vi "Day 6.vi"() -> ()   [LabVIEW 2019]
panel:
  out "Largest Finite Area":i16
  out "Filtered Closest Point Indices":i32[][](array[numeric])
  out "Closest Point Indices":i32[][](array[numeric])
  out "Distances":i32[][][](array[numeric])
  out "Min Values":i32[](array[numeric])
  out "Max Values":i32[](array[numeric])
  out "Coordinates":i32[][](array[numeric])
  in  "Error In":errorcluster
  in  "Use Example Input":bool
  in  "Example Input":string="1, 1\n1, 6\n8, 3\n3, 4\n5, 5\n8, 9\n"
  in  "Relative Path to Input File":string="Day 6\\Day 6 Raw Input.txt"
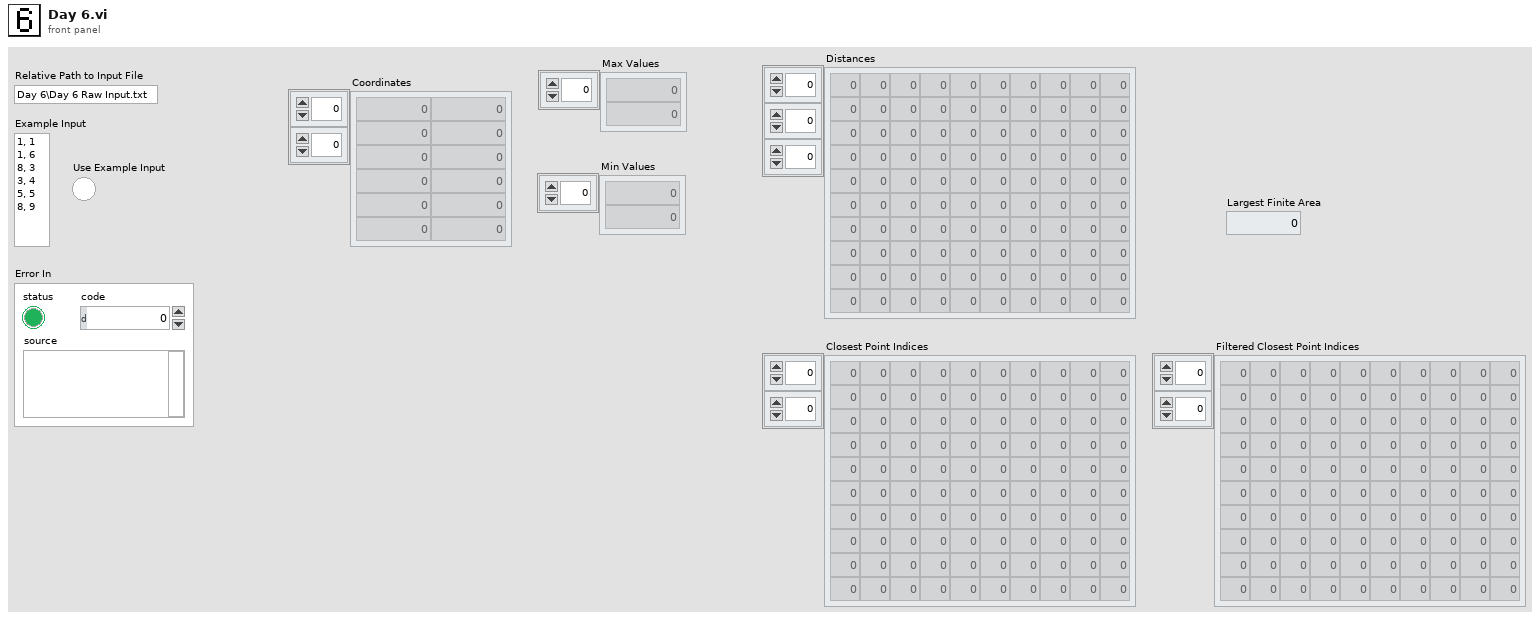
[diagram p1: front panel]
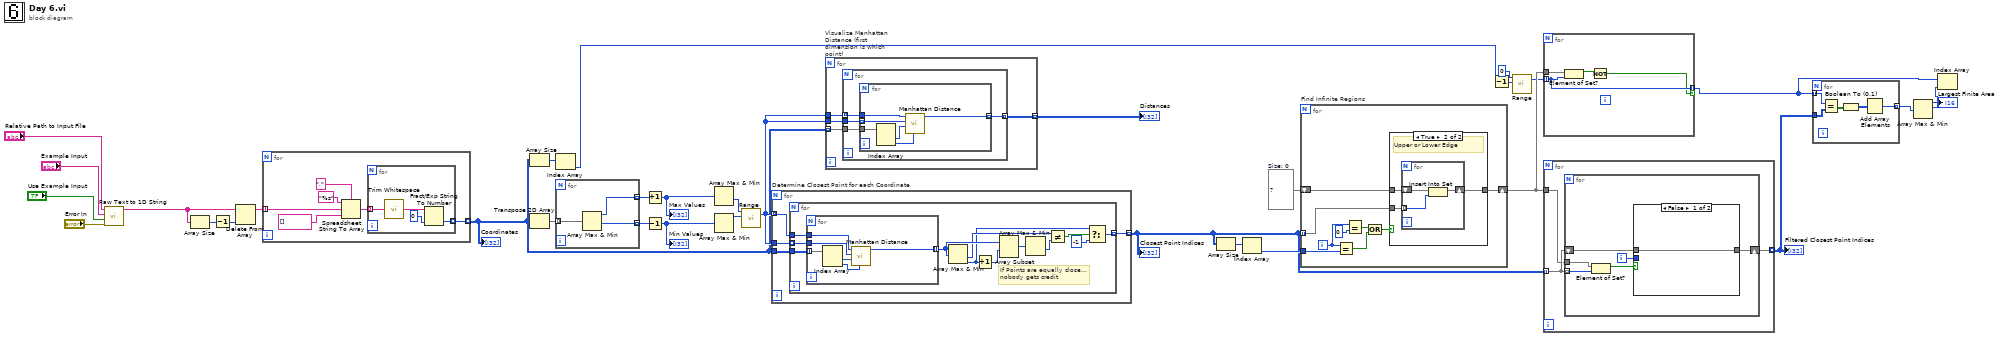
[diagram p0: block diagram]
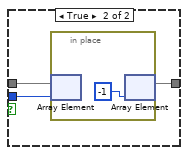
[diagram p2: hidden frame]
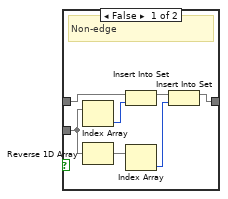
[diagram p3: hidden frame]
diagram:
  w14 = set{i32} {}  # Size: 0
  n1 = call "Raw Text to 1D String.vi"("Error In"="Error In", "Use Example Input"="Use Example Input", "Example Input"="Example Input", "Relative Path to Input File"="Relative Path to Input File") -> ("1D String Array"=w26:string[])  [unwired: 6 in, 1 out]
  n2 = Array Size(array=w26) -> (size(s)=w28:i32)
  n3 = Decrement(x=w28) -> (x-1=w27:i32)
  n4 = Delete From Array(array=w26, index=w27) -> (array with subset deleted=w25:string[])  [unwired: 1 in, 1 out]
  n5 = for {
    tunnel: w25 -> [w39] mode=indexing
    tunnel: [w34] -> w12 mode=indexing
    n6 = Spreadsheet String To Array(delimiter (Tab)="," ("delimiter"), format string="%s", spreadsheet string=w39, array type (2D Dbl)=string[] []) -> (array=w36:string[])
    n7 = for {
      tunnel: w36 -> [w43] mode=indexing
      tunnel: [w40] -> w34 mode=indexing
      n8 = call <vilib>:"Trim Whitespace.vi"("string"=w43) -> ("trimmed string"=w42:string)  [unwired: 1 in]
      n9 = Fract/Exp String To Number(string=w42, default (0 dbl)=0 ("default (0 DBL)")) -> (number=w40:i32)  [unwired: 2 in, 1 out]
    }
  }
  "Coordinates" <- w12
  n10 = Array Size(array=w12) -> (size(s)=w10:i32[])
  n11 = Transpose 2D Array(2D array=w12) -> (transposed array=w29:i32[][])
  n12 = Index Array(array=w10) -> (element=w9:i32)  [unwired: 1 in]
  n13 = for {
    tunnel: w29 -> [w46] mode=indexing
    tunnel: [w45] -> w23 mode=indexing
    tunnel: [w44] -> w24 mode=indexing
    n14 = Array Max & Min(array=w46) -> (max value=w45:i32, min value=w44:i32)  [unwired: 2 out]
  }
  n15 = Increment(x=w23) -> (x+1=w22:i32[])
  "Max Values" <- w22
  n16 = Decrement(x=w24) -> (x-1=w21:i32[])
  "Min Values" <- w21
  n17 = Array Max & Min(array=w22) -> (min value=w20:i32)  [unwired: 3 out]
  n18 = Array Max & Min(array=w21) -> (max value=w19:i32)  [unwired: 3 out]
  n19 = call "Range.vi"("y"=w19, "x"=w20) -> ("Range"=w17:i32[])  [unwired: 5 in]
  n20 = for "Determine Closest Point for each Coordinate" {
    tunnel: w17 -> [w49] mode=indexing
    tunnel: w17 -> [w50]
    tunnel: w12 -> [w48]
    tunnel: [w47] -> w13 mode=indexing
    n21 = for {
      tunnel: w50 -> [w61] mode=indexing
      tunnel: w49 -> [w60]
      tunnel: w48 -> [w62]
      tunnel: [w53] -> w47 mode=indexing
      # "If Points are equally close...\nnobody gets credit"
      n22 = for {
        tunnel: w62 -> [w68] mode=indexing
        tunnel: w61 -> [w64]
        tunnel: w60 -> [w65]
        tunnel: [w63] -> w59 mode=indexing
        n23 = Index Array(array=w68) -> (element #1=w67:i32, element #2=w66:i32)  [unwired: 2 in]
        n24 = call "Manhattan Distance.vi"("y 2"=w66, "x 2"=w67, "x"=w64, "y"=w65) -> ("Manhattan Distance"=w63:i32)  [unwired: 7 in]
      }
      n25 = Array Max & Min(array=w59) -> (min value=w57:i32, min index (indices)=w52:i32)  [unwired: 2 out]
      n26 = Increment(x=w52) -> (x+1=w51:i32)
      n27 = Array Subset(array=w59, index=w51) -> (w58:i32[])  [unwired: 1 in]
      n28 = Array Max & Min(array=w58) -> (min value=w56:i32)  [unwired: 3 out]
      n29 = Not Equal?(x=w57, y=w56) -> (x != y?=w55:bool)
      n30 = Select(t=w52, s=w55, f=-1) -> (s? t:f=w53:i32)
    }
  }
  "Closest Point Indices" <- w13
  n31 = for "Visualize Manhattan Distance (first dimension is which point)" {
    tunnel: w17 -> [w71]
    tunnel: w17 -> [w72]
    tunnel: w12 -> [w70] mode=indexing
    tunnel: [w69] -> w18 mode=indexing
    n32 = for {
      tunnel: w72 -> [w75]
      tunnel: w71 -> [w74] mode=indexing
      tunnel: w70 -> [w76]
      tunnel: [w73] -> w69 mode=indexing
      n33 = for {
        tunnel: w76 -> [w82]
        tunnel: w75 -> [w78] mode=indexing
        tunnel: w74 -> [w79]
        tunnel: [w77] -> w73 mode=indexing
        n34 = Index Array(array=w82) -> (element #1=w81:i32, element #2=w80:i32)  [unwired: 2 in]
        n35 = call "Manhattan Distance.vi"("y 2"=w80, "x 2"=w81, "x"=w78, "y"=w79) -> ("Manhattan Distance"=w77:i32)  [unwired: 7 in]
      }
    }
  }
  "Distances" <- w18
  n36 = Array Size(array=w13) -> (size(s)=w16:i32[])
  n37 = Index Array(array=w16) -> (element=w15:i32)  [unwired: 1 in]
  n38 = for "Find Infinite Regions" {
    tunnel: w13 -> [w86] mode=indexing
    tunnel: w15 -> [w88]
    shift-right: [w84] -> w8
    shift-left: w14 -> [w85]
    i -> [w89]
    n39 = Equal?(x=w89, y=w88) -> (x = y?=w91:bool)
    n40 = Equal?(x=w89, y=0) -> (x = y?=w90:bool)
    n41 = Or(x=w90, y=w91) -> (x .or. y?=w83:bool)
    n42 = case shown="True" w83 {
      tunnel: w86 -> [w95 w101]
      tunnel: w85 -> [w98 w100]
      tunnel: [w96 w99] -> w84
      frame False {
        # "Non-edge"
        n43 = Index Array(array=w95) -> (element=w93:i32)  [unwired: 1 in]
        n44 = Reverse 1D Array(array=w95) -> (reversed array=w94:i32[])
        n45 = Insert Into Set(10:w93, 11:w98) -> (3:w97:set{i32})  [unwired: 1 out]
        n46 = Index Array(array=w94) -> (element=w92:i32)  [unwired: 1 in]
        n47 = Insert Into Set(10:w92, 11:w97) -> (3:w96:set{i32})  [unwired: 1 out]
      }
      frame True {
        # "Upper or Lower Edge"
        n48 = for {
          tunnel: w101 -> [w102] mode=indexing
          shift-right: [w103] -> w99
          shift-left: w100 -> [w104]
          n49 = Insert Into Set(10:w102, 11:w104) -> (3:w103:set{i32})  [unwired: 1 out]
        }
      }
    }
  }
  n50 = Decrement(x=w9) -> (x-1=w2:i32)
  n51 = call "Range.vi"("y"=w2, "x"=0) -> ("Range"=w7:i32[])  [unwired: 5 in]
  n52 = for {
    tunnel: w8 -> [w108]
    tunnel: w7 -> [w107] mode=indexing
    tunnel: [w107] -> w1 mode=indexing if=w105
    n53 = Element of Set?(10:w107, 11:w108) -> (3:w106:bool)
    n54 = Not(x=w106) -> (.not. x?=w105:bool)
  }
  n55 = for {
    tunnel: w13 -> [w111] mode=indexing
    tunnel: [w110] -> w6 mode=indexing
    tunnel: w8 -> [w109]
    n56 = for {
      tunnel: w111 -> [w113] mode=indexing
      shift-right: [w115] -> w110
      shift-left: w111 -> [w117]
      tunnel: w109 -> [w114]
      i -> [w116]
      n57 = Element of Set?(10:w113, 11:w114) -> (3:w112:bool)
      n58 = case shown="False" w112 {
        tunnel: w117 -> [w118 w121]
        tunnel: w116 -> [_ w120]
        tunnel: [w118 w119] -> w115
        frame False {
        }
        frame True {
          n59 = in-place {
            n60 = in-place-array #1(w121, w120) -> ()  [unwired: 1 out]
            n61 = in-place-array #1(-1 ("f")) -> (w119:i32[])  [unwired: 1 out]
          }
        }
      }
    }
  }
  "Filtered Closest Point Indices" <- w6
  n62 = for {
    tunnel: w1 -> [w127] mode=indexing
    tunnel: w6 -> [w126]
    tunnel: [w123] -> w5 mode=indexing
    n63 = Equal?(x=w127, y=w126) -> (x = y?=w125:bool[][])
    n64 = Boolean To (0,1)(Boolean=w125) -> (0, 1=w124:i16[][])
    n65 = Add Array Elements(numeric array=w124) -> (sum=w123:i16)
  }
  n66 = Array Max & Min(array=w5) -> (max value=→"Largest Finite Area":i16, max index (indices)=w4:i32)  [unwired: 2 out]
  n67 = Index Array(array=w1, index=w4) -> ()  [unwired: 1 out]
